vi "Tarea 1.vi"() -> ()   [LabVIEW 2019]
panel:
  in  "Stop VI":bool
  out "Time has elapsed":bool
  out "Elapsed Time":dbl
  in  "Auto Reset":bool
  in  "Reset":bool
  in  "Time Timer":dbl
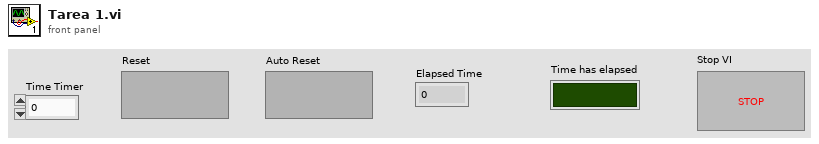
[diagram p1: front panel]
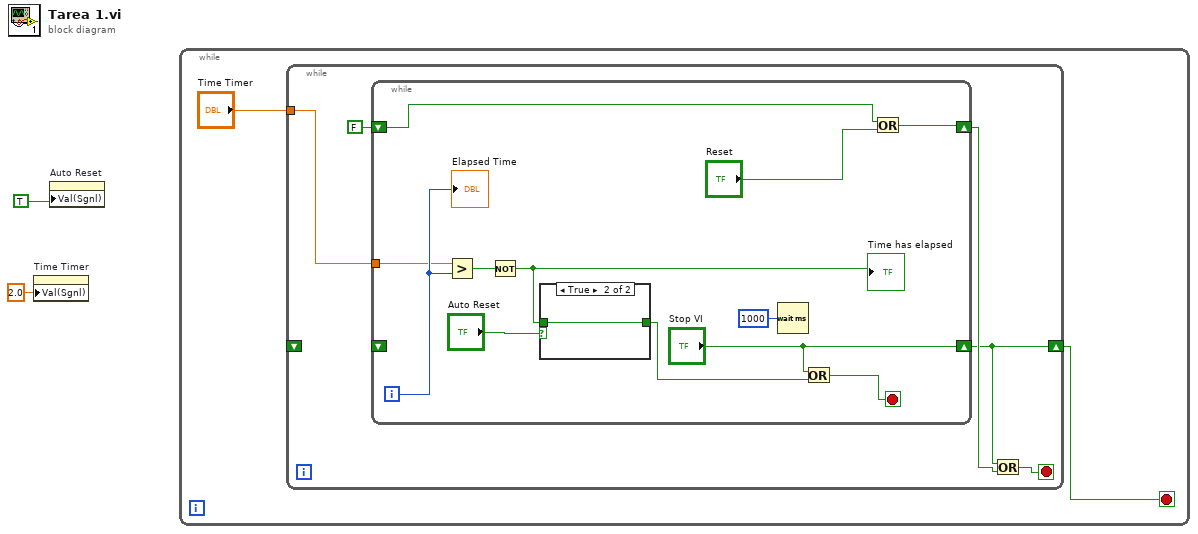
[diagram p0: block diagram]
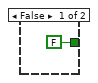
[diagram p2: hidden frame]
diagram:
  n1 = property on="Time Timer" class="DigNum (strict)"("Val(Sgnl)"=2.0 ("Value (Signaling)")) -> ()  [unwired: 2 in, 2 out]
  n2 = property on="Auto Reset" class="Bool (strict)"("Val(Sgnl)"=TRUE ("Value (Signaling)")) -> ()  [unwired: 2 in, 2 out]
  n3 = while {
    stop <- w3 stop-if-true
    n4 = while {
      tunnel: "Time Timer" -> [w9]
      shift-right: [w6] -> w3
      shift-left: _ -> [_]
      stop <- w8 stop-if-true
      n5 = while {
        tunnel: w9 -> [w17]
        shift-right: ["Stop VI"] -> w6
        shift-left: _ -> [_]
        shift-right: [w12] -> w7
        shift-left: FALSE -> [w10]
        i -> [w20]
        stop <- w19 stop-if-true
        n6 = Greater?(x=w17, y=w20) -> (0:w16:bool)
        n7 = Not(x=w16) -> (.not. x?=w14:bool)
        "Time has elapsed" <- w14
        n8 = case shown="True" "Auto Reset" {
          tunnel: [FALSE w23] -> w13
          tunnel: w14 -> [_ w23]
          frame False {
          }
          frame True {
          }
        }
        n9 = Wait (ms)(milliseconds to wait=u32 1000) -> ()  [unwired: 1 out]
        n10 = Or(x="Stop VI", y=w13) -> (x .or. y?=w19:bool)
        n11 = Or(x=w10, y="Reset") -> (x .or. y?=w12:bool)
        "Elapsed Time" <- w20
      }
      n12 = Or(x=w6, y=w7) -> (x .or. y?=w8:bool)
    }
  }
